vi "消息提示.vi"(7 "设置":string[](array[string]), 8 "被测幅值":dbl[](array[numeric]), 9 "参考幅值":dbl format="%.2p", 10 "参数":string(combo)="参考灵敏度") -> ()   [LabVIEW 2015]
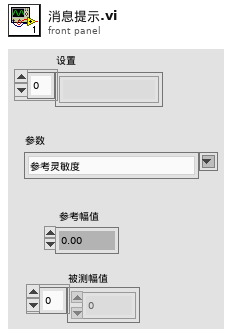
[diagram p1: front panel]
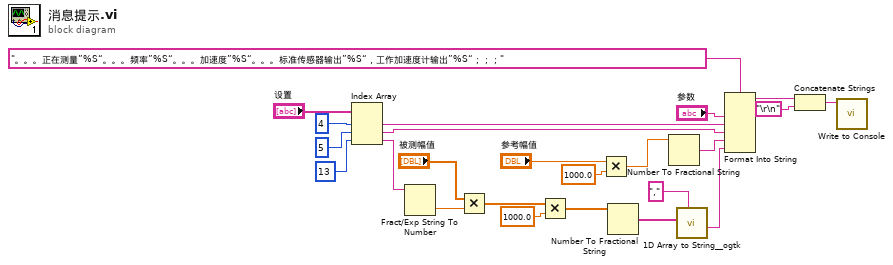
[diagram p0: block diagram]
diagram:
  n1 = Index Array(array="设置", index #1=4 ("索引"), index #2=5 ("索引"), index #3=13 ("索引")) -> (element #1=w20:string, element #2=w11:string, element #3=w12:string)
  n2 = Fract/Exp String To Number(string=w12) -> (number=w18:dbl)  [unwired: 3 in, 1 out]
  n3 = Multiply(x="被测幅值", y=w18) -> (x*y=w17:dbl[])
  n4 = Multiply(x=w17, y=1000.0) -> (x*y=w8:dbl[])
  n5 = Multiply(x="参考幅值", y=1000.0) -> (x*y=w14:dbl)
  n6 = Number To Fractional String(number=w8) -> (F-format string=w3:string[])  [unwired: 3 in]
  n7 = Number To Fractional String(number=w14) -> (F-format string=w9:string)  [unwired: 3 in]
  n8 = call <userlib>:"1D Array to String__ogtk.vi"("delimiter (Tab)"=",", "Array of Strings"=w3) -> ("delimited string"=w1:string)  [unwired: 9 in]
  n9 = Format Into String(format string="。。。正在测量”%S“。。。频率”%S“。。。加速度”%S“。。。标准传感器输出”%S“，工作加速度计输出”%S“；；；" ("分隔符(Tab)"), "参数", w20, w11, w9, w1) -> (resulting string=w5:string)  [unwired: 2 in, 1 out]
  n10 = Concatenate Strings(w5, "\r\n") -> (w6:string)
  n11 = call "Write to Console.vi"("Input"=w6) -> ()  [unwired: 10 in, 1 out]
